vi "Micro-PL Drive Calibration v10.6.1.vi"() -> ()   [LabVIEW 2010]
uses:
  <vilib>/Utility/miscctls.llb/LVPointTypeDef.ctl
  <vilib>/Utility/file.llb/Write To Spreadsheet File (DBL).vi
panel:
  in  "Voltage Stop":dbl=130.0 caption="Stop (V)" min=-20.0 max=130.0 step=0.001
  in  "Voltage Start":dbl=-20.0 caption="Start (V)" min=-20.0 max=130.0 step=0.001
  in  "Drive Connection":refnum<visa-resource-name>="COM6" caption="Drive COM Port"
  in  "Snapshot Folder":path=path "C:/Users/WET-KORR/Desktop/Screenshots"
  in  "Camera Name":string="HD USB Camera"
  in  "Start":bool
  out "Voltages":ext[][](array[numeric])
  out "Current Voltage":ext caption="Current (V)" format="%.3f"
  in  "Axis":u16(ring) items=["X", "Y", "Z"]
  out "Progress":u8(slide) max=10 scale=0.0..100.0
  in  "Exit":bool
  in  "Voltage Step":dbl=0.01 caption="Step (V)" min=0.001 max=5.0 step=0.001
  # "Drive Calibration"
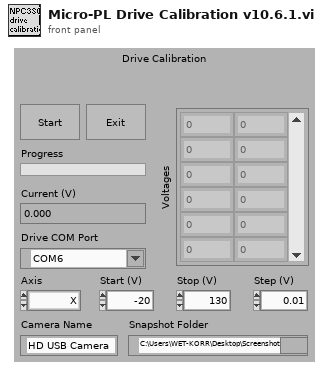
[diagram p1: front panel]
types:
  T1 = typedef "LVPointTypeDef.ctl" = cluster{"Horizontal":i16, "Vertical":i16}
  T2 = typedef "NPC3SG Current Voltages v10.6.1.ctl" = cluster{"Drive X Voltage":dbl, "Drive Y Voltage":dbl, "Drive Z Voltage":dbl}
  T3 = enum32{"invalid app kind", "Development System", "Run Time System", "Student Edition", "Embedded LabVIEW", "Evaluation", "Custom"}
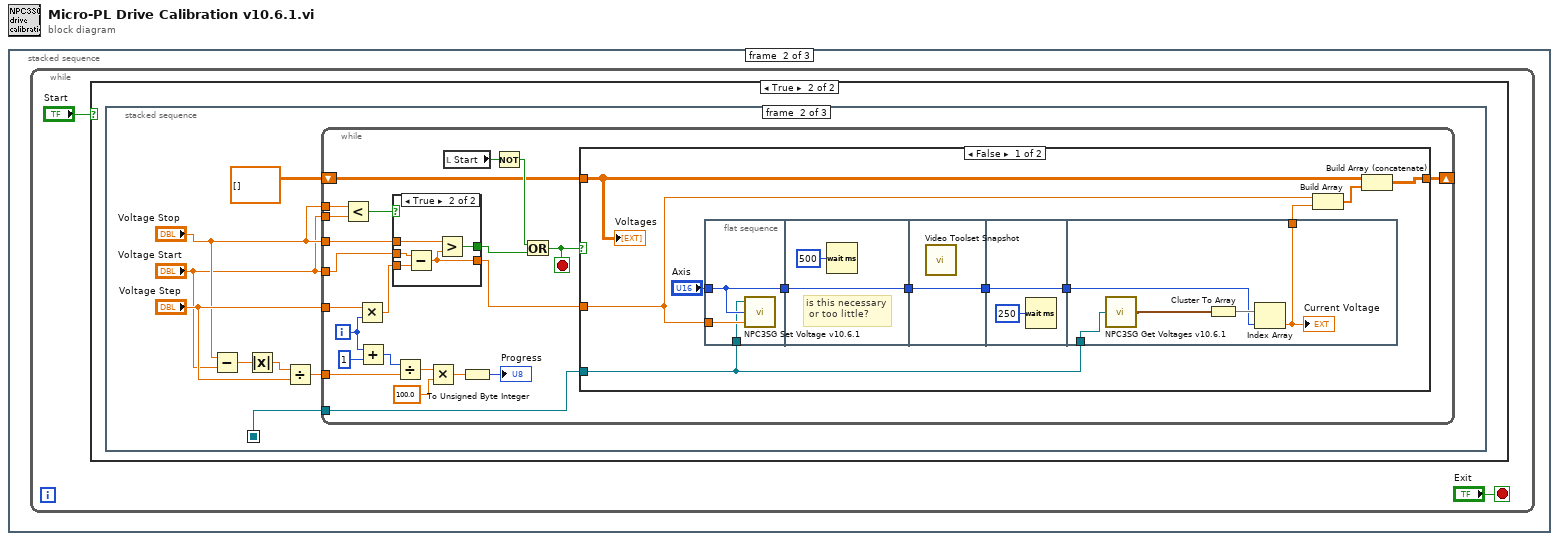
[diagram p0: block diagram]
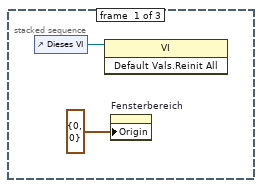
[diagram p2: hidden frame]
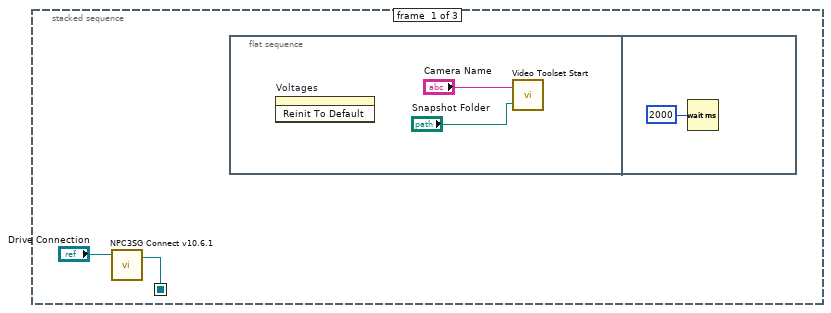
[diagram p4: hidden frame]
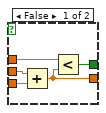
[diagram p5: hidden frame]
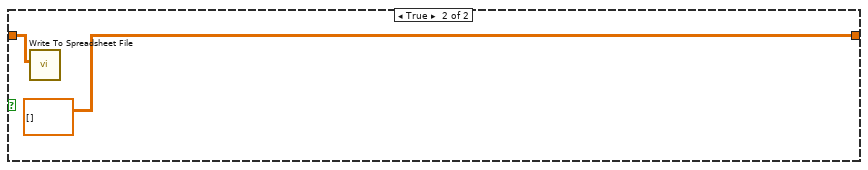
[diagram p6: hidden frame]
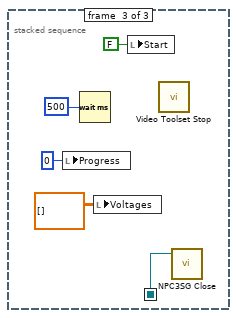
[diagram p7: hidden frame]
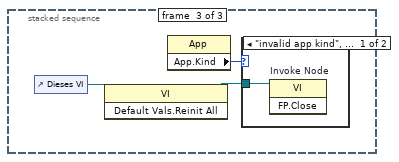
[diagram p8: hidden frame]
diagram:
  n1 = stacked-sequence {
    frame #0 {
      n2 = control-ref of="Dieses VI"() -> (w1:refnum<vi>)
      n3 = invoke class="VI" method="Default Vals.Reinit All"(reference=w1) -> ()  [unwired: 2 in, 3 out]
      n4 = property on="Fensterbereich" class="Pane"("Origin"=T1 {"Horizontal"=0, "Vertical"=0}) -> ()  [unwired: 2 in, 2 out]
    }
    frame #1 {
      n5 = while {
        stop <- "Exit" stop-if-true
        n6 = case shown="True" "Start" {
          frame False {
          }
          frame True {
            n7 = stacked-sequence {
              seq-local: [w6 _ _] -> [_ w14 w77]
              frame #0 {
                n8 = call "NPC3SG Connect v10.6.1.vi"("Drive Port"="Drive Connection") -> ("Drive Visa Name"=w6:refnum<visa-resource-name>)  [unwired: 2 in, 1 out]
                n9 = flat-sequence {
                  frame #0 {
                    n10 = invoke on="Voltages" class="Arr (strikt)" method="Reinit To Default"() -> ()  [unwired: 3 in, 3 out]
                    n11 = call "Video Toolset Start.vi"("Snapshot Folder"="Snapshot Folder", "Camera Name"="Camera Name") -> ()  [unwired: 1 in]
                  }
                  frame #1 {
                    n12 = Wait (ms)(milliseconds to wait=u32 2000 ("Timer-Wert (ms)")) -> ()  [unwired: 1 out]
                  }
                }
              }
              frame #1 {
                n13 = Subtract(x="Voltage Stop", y="Voltage Start") -> (x-y=w13:dbl)
                n14 = Absolute Value(x=w13) -> (abs(x)=w12:dbl)
                n15 = Divide(x=w12, y="Voltage Step") -> (x/y=w16:dbl)
                n16 = while {
                  tunnel: "Voltage Start" -> [w27]
                  tunnel: "Voltage Step" -> [w24]
                  tunnel: "Voltage Stop" -> [w31]
                  tunnel: w16 -> [w33]
                  tunnel: w14 -> [w19]
                  shift-right: [w18] -> _
                  shift-left: dbl[][] [] -> [w26]
                  tunnel: "Voltage Stop" -> [w22]
                  tunnel: "Voltage Start" -> [w21]
                  i -> [w25]
                  stop <- w38 stop-if-true
                  n17 = Less?(x=w22, y=w21) -> (x < y?=w20:bool)
                  n18 = Multiply(x=w24, y=w25) -> (x*y=w23:dbl)
                  n19 = Add(x=w25, y=1) -> (x+y=w34:i32)
                  n20 = case shown="True" w20 {
                    tunnel: [w45 w50] -> w40
                    tunnel: w31 -> [w41 w49]
                    tunnel: [w44 w48] -> w30
                    tunnel: w27 -> [w43 w47]
                    tunnel: w23 -> [w42 w46]
                    frame False {
                      n21 = Add(x=w43, y=w42) -> (x+y=w44:dbl)
                      n22 = Less?(x=w41, y=w44) -> (x < y?=w45:bool)
                    }
                    frame True {
                      n23 = Subtract(x=w47, y=w46) -> (x-y=w48:dbl)
                      n24 = Greater?(x=w49, y=w48) -> (0:w50:bool)
                    }
                  }
                  n25 = Divide(x=w34, y=w33) -> (x/y=w39:dbl)
                  n26 = Multiply(x=w39, y=100.0) -> (x*y=w37:dbl)
                  n27 = local read "Start"() -> (w29:bool)
                  n28 = To Unsigned Byte Integer(number=w37) -> (unsigned 8bit integer=→"Progress":u8)
                  n29 = Not(x=w29) -> (.not. x?=w28:bool)
                  n30 = Or(x=w28, y=w40) -> (x .or. y?=w38:bool)
                  n31 = case shown="False" w38 {
                    tunnel: w30 -> [w51 _]
                    tunnel: w26 -> [w52 w76]
                    tunnel: [w53 dbl[][] []] -> w18
                    tunnel: w19 -> [w54 _]
                    frame False {
                      n32 = flat-sequence {
                        tunnel: w51 -> [w63]
                        tunnel: "Axis" -> [w64]
                        tunnel: [w64] -> w61
                        tunnel: w54 -> [w62]
                        tunnel: w61 -> [w66]
                        tunnel: [w66] -> w60
                        tunnel: w60 -> [w67]
                        tunnel: [w67] -> w59
                        tunnel: [w69] -> w58
                        tunnel: w59 -> [w69]
                        tunnel: w58 -> [w70]
                        tunnel: w54 -> [w71]
                        tunnel: [w74] -> w56
                        frame #0 {
                          n33 = call "NPC3SG Set Voltage v10.6.1.vi"("Voltage"=w63, "Axis"=w64, "Drive Visa Name"=w62) -> ()  [unwired: 1 in, 1 out]
                        }
                        frame #1 {
                          # "is this necessary\n or too little?"
                          n34 = Wait (ms)(milliseconds to wait=u32 500) -> ()  [unwired: 1 out]
                        }
                        frame #2 {
                          n35 = call "Video Toolset Snapshot.vi"() -> ()  [unwired: 12 in]
                        }
                        frame #3 {
                          n36 = Wait (ms)(milliseconds to wait=u32 250) -> ()  [unwired: 1 out]
                        }
                        frame #4 {
                          n37 = call "NPC3SG Get Voltages v10.6.1.vi"("Drive Visa Name"=w71) -> ("Drive Current Voltages"=w72:T2)
                          n38 = Cluster To Array(cluster=w72) -> (array=w73:dbl[])
                          n39 = Index Array(array=w73, index=w70) -> (element=w74:dbl)
                          "Current Voltage" <- w74
                        }
                      }
                      n40 = Build Array(w51, w56) -> (w55:dbl[])
                      n41 = Build Array (concatenate)(w52, w55) -> (w53:dbl[][])
                      "Voltages" <- w52
                    }
                    frame True {
                      n42 = call-poly <vilib>:"Write To Spreadsheet File.vi"("2D data"=w76) -> ()  [unwired: 7 in, 1 out]
                    }
                  }
                }
              }
              frame #2 {
                n43 = local write "Progress"(u8 0 ("Progress")) -> ()
                n44 = Wait (ms)(milliseconds to wait=u32 500 ("Timer-Wert (ms)")) -> ()  [unwired: 1 out]
                n45 = local write "Voltages"(ext[][] [] ("Voltages")) -> ()
                n46 = local write "Start"(FALSE ("Start")) -> ()
                n47 = call "Video Toolset Stop.vi"() -> ()  [unwired: 3 in]
                n48 = call "NPC3SG Close.vi"("Drive Visa Name"=w77) -> ()  [unwired: 4 in]
              }
            }
          }
        }
      }
    }
    frame #2 {
      n49 = control-ref of="Dieses VI"() -> (w84:refnum<vi>)
      n50 = invoke class="VI" method="Default Vals.Reinit All"(reference=w84) -> (reference out=w82:refnum<vi>)  [unwired: 2 in, 2 out]
      n51 = property class="App"() -> ("App.Kind"=w83:T3)  [unwired: 2 in, 2 out]
      n52 = case shown="\"invalid app kind\", Default" w83 {
        tunnel: w82 -> [w85 _]
        frame "invalid app kind", Default {
          n53 = invoke on="Invoke Node" class="VI" method="FP.Close"(reference=w85) -> ()  [unwired: 2 in, 3 out]
        }
        frame "Development System" {
        }
      }
    }
  }
